vi "Read as Pixmap Mono12.vi"(4 "Mask (Empty: None)":u8[](array[numeric]), 6 "Colours (Empty: Use Greyscale)":u32[](array[numeric]), 7 "Top Left Point (0,0)":T2, 8 "error in (no error)":errorcluster, 11 "Buffer in":refnum<class "Buffer.lvclass">) -> (0 "error out":errorcluster, 2 "Image Data":T1, 3 "Buffer":refnum<class "Buffer.lvclass">)   [LabVIEW 2020, in "Buffer.lvclass"]
doc: "Read the buffer data assuming it is in the Mono 12 pixel format and return it as a LabVIEW Flattened Pixmap."
uses:
  Buffer.lvclass
  Picture Top Left Point Offset.ctl
  <vilib>/picture/picture.llb/imagedata.ctl
  Pixel Formats.ctl
  Buffer.lvclass/Buffer.ctl
  <vilib>/Utility/error.llb/Error Cluster From Error Code.vi
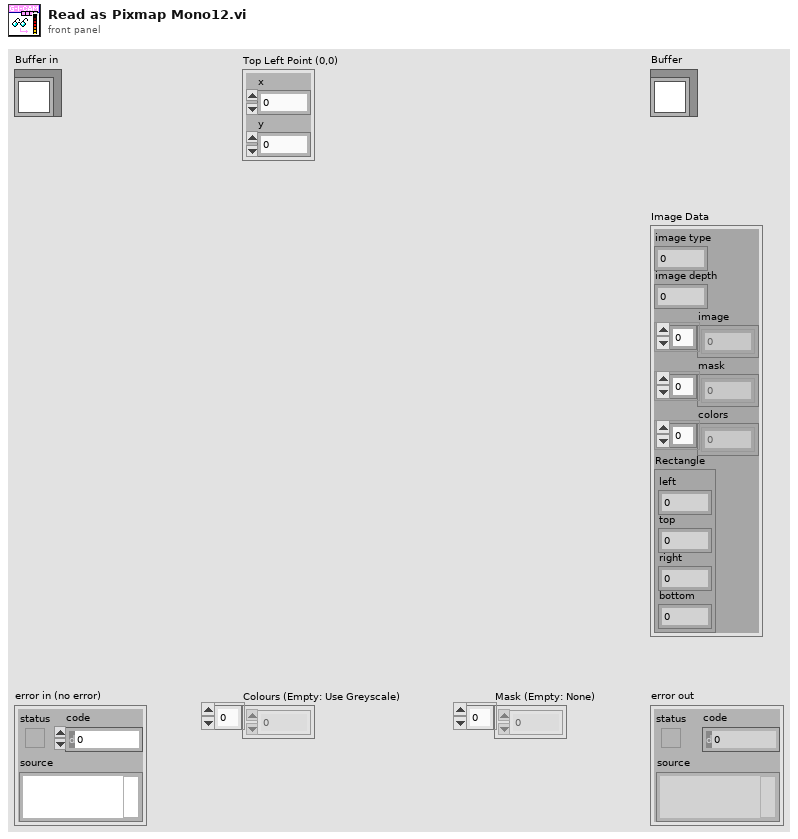
[diagram p1: front panel]
types:
  T1 = typedef "imagedata.ctl" = cluster{"image type":i32, "image depth":i32, "image":u8[], "mask":u8[], "colors":u32[], "Rectangle":cluster{"left":i16, "top":i16, "right":i16, "bottom":i16}}
  T2 = typedef "Buffer.lvclass/Picture Top Left Point Offset.ctl" = cluster{"x":i16, "y":i16}
  T3 = typedef "Buffer.lvclass/Pixel Formats.ctl" = enum16{"mono8", "mono10", "mono10p", "mono12", "mono12p", "mono14", "mono14p", "mono16", "RGB8", "BGR8"}
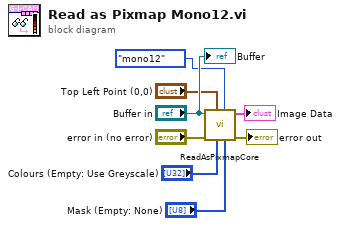
[diagram p0: block diagram]
diagram:
  n1 = call "ReadAsPixmapCore.vi"("mask"="Mask (Empty: None)", "Pixel Formats"=Pixel_Formats."mono12", "colours"="Colours (Empty: Use Greyscale)", "Top Left Point"="Top Left Point (0,0)", "error in (no error)"="error in (no error)", "Buffer In"="Buffer in") -> ("error out"=→"error out":errorcluster, "pixmap"=→"Image Data":T1)  [unwired: 4 in]
  "Buffer" <- "Buffer in"
